vi "Calculate Delta.vi"(10 "Last Time":dbl format="%_19f", 11 "Property":sgl) -> (3 "Delta":sgl)   [LabVIEW 2021]
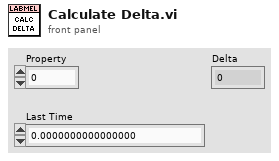
[diagram p1: front panel]
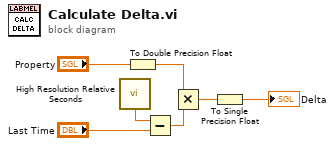
[diagram p0: block diagram]
diagram:
  n1 = call <vilib>:"High Resolution Relative Seconds.vi"() -> ("relative seconds"=w7:dbl)
  n2 = To Double Precision Float(number="Property") -> (double precision float=w5:dbl)
  n3 = Subtract(x=w7, y="Last Time") -> (x-y=w6:dbl)
  n4 = Multiply(x=w5, y=w6) -> (x*y=w2:dbl)
  n5 = To Single Precision Float(number=w2) -> (single precision float=→"Delta":sgl)
